vi "Adquisicion.vi"(1 "Aviso no detección":string) -> (0 "String":string)   [LabVIEW 2015]
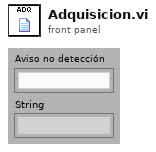
[diagram p1: front panel]
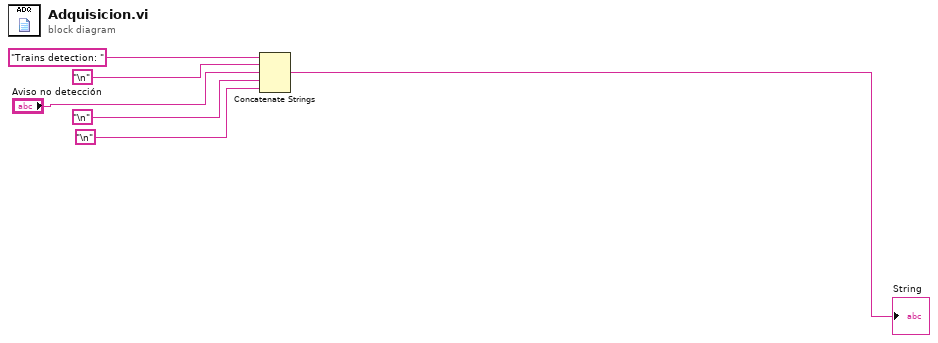
[diagram p0: block diagram]
diagram:
  n1 = Concatenate Strings("Trains detection: ", "\n", "Aviso no detección", "\n", "\n") -> (→"String":string)
